vi "SelectStriptestProber.vi"(8 "error in (no error)":errorcluster) -> (0 "error out":errorcluster, 3 "ProbeStationControl out":refnum<class "ProbeStationControl.lvclass">)   [LabVIEW 2018, in "ProbeStationControl.lvclass"]
uses:
  ProbeStationControl.lvclass
  SemiProbe/SemiProbe.lvclass
  Alessi Rel-6100/AlessiRel6100.lvclass
  C:/Users/veral/Documents/itk-strip-sensor-qc/LabVIEW 2013/InstrControl/ProbeStationControl/ProbeStationControl.lvclass
panel:
  out "Tab Control":enum32{"Select Prober", "Load sensor"}(tab)
  in  "Select Probestation":enum16{"Alessi REL-6100", "SemiProbe"}(ring)
  in  "Cancel Button":bool
  in  "Continue":bool
  in  "Move down?":bool caption="Chuck\nDOWN"
  in  "Eject Button":bool
  in  "Continue 2":bool
  in  "Cancel Button 2":bool
  # "Klick to:"
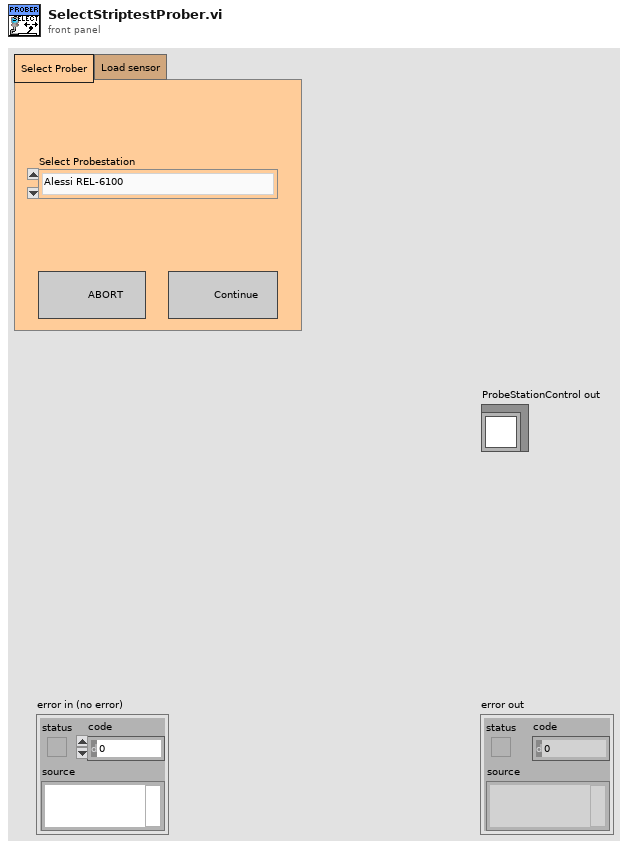
[diagram p1: front panel]
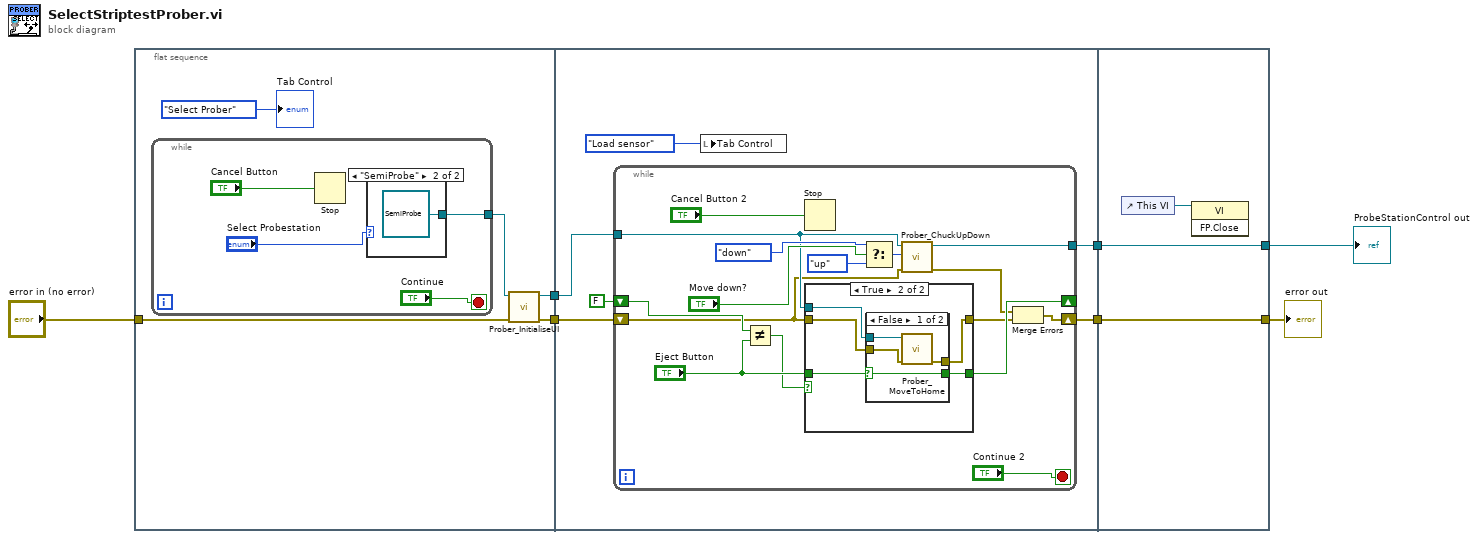
[diagram p0: block diagram]
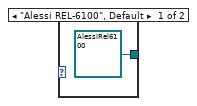
[diagram p2: hidden frame]
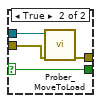
[diagram p4: hidden frame]
diagram:
  n1 = flat-sequence {
    tunnel: "error in (no error)" -> [w9]
    tunnel: [w8] -> w6
    tunnel: [w11] -> w5
    tunnel: w6 -> [w22]
    tunnel: w5 -> [w23]
    tunnel: [w21] -> w2
    tunnel: [w19] -> w1
    tunnel: [w57] -> w3
    tunnel: [w58] -> w4
    tunnel: w2 -> [w58]
    tunnel: w1 -> [w57]
    frame #0 {
      n2 = while {
        tunnel: [w13] -> w10
        stop <- "Continue" stop-if-true
        n3 = Stop(stop? (T)="Cancel Button") -> ()
        n4 = case shown="\"SemiProbe\"" "Select Probestation" {
          tunnel: [refnum<class "AlessiRel6100.lvclass"> refnum ("AlessiRel6100.lvclass") refnum<class "SemiProbe.lvclass"> refnum ("SemiProbe.lvclass")] -> w13
          frame "Alessi REL-6100", Default {
          }
          frame "SemiProbe" {
          }
        }
      }
      n5 = call-dynamic "Prober_InitialiseUI.vi"("error in (no error)"=w9, "ProbeStationControl in"=w10) -> ("error out"=w8:errorcluster, "ProbeStationControl out"=w11:refnum<class "ProbeStationControl.lvclass">)  [unwired: 7 in, 1 out]
      "Tab Control" <- enum32{"Select Prober", "Load sensor"}."Select Prober" ("Tab Control")
    }
    frame #1 {
      n6 = while {
        tunnel: w23 -> [w36]
        shift-right: [w30] -> _
        shift-left: FALSE -> [w34]
        shift-right: [w26] -> w21
        shift-left: w22 -> [w29]
        tunnel: [w25] -> w19
        stop <- "Continue 2" stop-if-true
        n7 = Not Equal?(x=w34, y="Eject Button") -> (x != y?=w33:bool)
        n8 = Stop(stop? (T)="Cancel Button 2") -> ()
        n9 = case shown="True" w33 {
          tunnel: w36 -> [_ w47]
          tunnel: "Eject Button" -> [w42 w46]
          tunnel: [w42 w45] -> w30
          tunnel: w29 -> [w41 w44]
          tunnel: [w41 w43] -> w27
          frame False {
          }
          frame True {
            n10 = case shown="False" w46 {
              selector: w46 -> [w50 w54]
              tunnel: w47 -> [w51 w55]
              tunnel: [w50 w54] -> w45
              tunnel: w44 -> [w49 w53]
              tunnel: [w48 w52] -> w43
              frame False {
                n11 = call-dynamic "Prober_MoveToHome.vi"("error in (no error)"=w49, "ProbeStationControl in"=w51) -> ("error out"=w48:errorcluster)  [unwired: 8 in, 1 out]
              }
              frame True {
                n12 = call-dynamic "Prober_MoveToLoad.vi"("error in (no error)"=w53, "ProbeStationControl in"=w55) -> ("error out"=w52:errorcluster)  [unwired: 8 in, 1 out]
              }
            }
          }
        }
        n13 = Select(t=enum16{"up", "down"}."down" ("Direction"), s="Move down?", f=enum16{"up", "down"}."up" ("Direction")) -> (s? t:f=w37:enum16{"up", "down"})
        n14 = call-dynamic "Prober_ChuckUpDown.vi"("error in (no error)"=w29, "Direction"=w37, "ProbeStationControl in"=w36) -> ("error out"=w28:errorcluster, "ProbeStationControl out"=w25:refnum<class "ProbeStationControl.lvclass">)  [unwired: 6 in, 1 out]
        n15 = Merge Errors(w28, w27) -> (w26:errorcluster)
      }
      n16 = local write "Tab Control"(enum32{"Select Prober", "Load sensor"}."Load sensor" ("Tab Control")) -> ()
    }
    frame #2 {
      n17 = control-ref of="This VI"() -> (w56:refnum<vi>)
      n18 = invoke class="VI" method="FP.Close"(reference=w56) -> ()  [unwired: 2 in, 3 out]
    }
  }
  "ProbeStationControl out" <- w3
  "error out" <- w4
